vi "get_data.vi"(0 "HGF_NetworkData":refnum<class "HGF_NetworkVisitor.lvclass">, 5 "error in (no error)":errorcluster) -> (14 "dup HGF_NetworkData":refnum<class "HGF_NetworkVisitor.lvclass">, 16 "data":variant, 17 "no link":bool, 19 "error out":errorcluster)   [LabVIEW 2014, in "HGF_BaseClasses.lvlib" / "HGF_NetworkVisitor.lvclass"]
uses:
  HGF_NetworkVisitor.lvclass
  HGF_PVSubscriber/HGF_PVSubscriber.lvclass
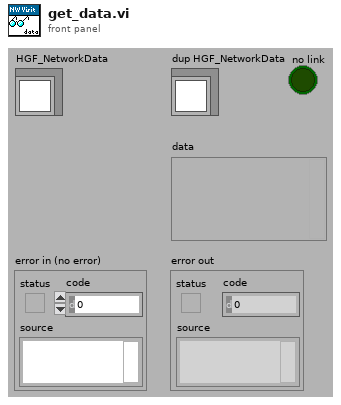
[diagram p1: front panel]
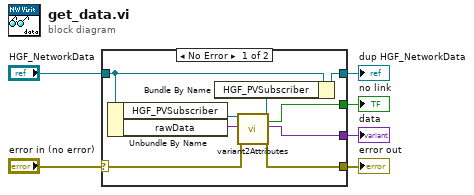
[diagram p0: block diagram]
diagram:
  n1 = case shown="No Error" "error in (no error)" {
    selector: "error in (no error)" -> [w9 w16]
    tunnel: [w8 w16] -> w5
    tunnel: [w11 w17] -> w3
    tunnel: "HGF_NetworkData" -> [w12 w17]
    tunnel: [w13 _] -> w2
    tunnel: [w7 _] -> w1
    frame No Error {
      n2 = Unbundle By Name(w12) -> ("HGF_PVSubscriber"=w15:refnum<class "HGF_PVSubscriber.lvclass">, "rawData"=w14:variant)
      n3 = call-dynamic "variant2Attributes.vi"("HGV_PVBase"=w15, "rawData"=w14, "error in (no error)"=w9) -> ("HGV_PVBase"=w10:refnum<class "HGF_PVSubscriber.lvclass">, "no link"=w7:bool, "Parameter"=w13:variant, "error out"=w8:errorcluster)  [unwired: 1 in, 12 out]
      n4 = Bundle By Name(cluster=w12, "HGF_PVSubscriber"=w10) -> (w11:refnum<class "HGF_NetworkVisitor.lvclass">)
    }
    frame Error {
    }
  }
  "error out" <- w5
  "dup HGF_NetworkData" <- w3
  "data" <- w2
  "no link" <- w1
